vi "Self Queue Alias.vi"(11 "Queue jettl in":refnum<class "Queue jettl.lvclass">) -> (2 "Self Queue Alias":string)   [LabVIEW 2021, in "jettl.lvlib" / "Queue jettl.lvclass"]
uses:
  Queue jettl.lvclass
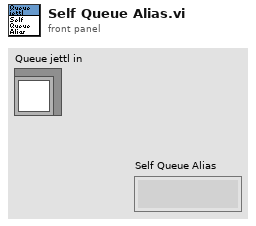
[diagram p1: front panel]
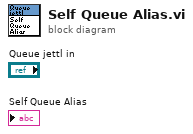
[diagram p0: block diagram]
diagram:
